vi "Poll For Jobs.vi"(8 "Error In":errorcluster, 10 "Job Queue WaitTime (5)":i32=5, 11 "VIChallenge Config in":T2) -> (0 "Error Ou":errorcluster, 2 "Worker State":T1, 3 "VIChallenge Config out":T2)   [LabVIEW 2013, in "VIChallenge.lvlib"]
uses:
  <vilib>/LabVIEW Hacker/VIChallenge/VIChallenge.lvlib
  <vilib>/LabVIEW Hacker/VIChallenge/Private/Type Defs/VIChallenge Config.ctl
  <vilib>/National Instruments/NI Amazon Web Services (AWS) Toolkit for LabVIEW/SQS/VI Source/AWS SQS Class/AWS_SQS.lvclass
  <vilib>/National Instruments/NI Amazon Web Services (AWS) Toolkit for LabVIEW/AWS Core Lib/VI Source/Typedefs/AWS_AWS Credentials.ctl
  <vilib>/LabVIEW Hacker/VIChallenge/Private/Type Defs/JSON_job.ctl
  <vilib>/addons/database/Connection.llb/Conn ObjectReference.ctl
  <vilib>/LabVIEW Hacker/VIChallenge/Private/Grader/Type Defs/Challenge.ctl
  <vilib>/LabVIEW Hacker/VIChallenge/Public/Worker State.ctl
  <vilib>/National Instruments/NI Amazon Web Services (AWS) Toolkit for LabVIEW/SQS/VI Source/Public Typedefs/AWS_SQS ReceiveMessage.ctl
  <vilib>/National Instruments/NI Amazon Web Services (AWS) Toolkit for LabVIEW/SQS/VI Source/Public Typedefs/AWS_SQS Queue Name and Account Number.ctl
  <vilib>/National Instruments/NI Amazon Web Services (AWS) Toolkit for LabVIEW/SQS/VI Source/AWS_SQS.lvlib
  <vilib>/National Instruments/NI Amazon Web Services (AWS) Toolkit for LabVIEW/AWS Core Lib/VI Source/AWS_Core.lvlib
  <vilib>/addons/database/NI_Database_API.lvlib
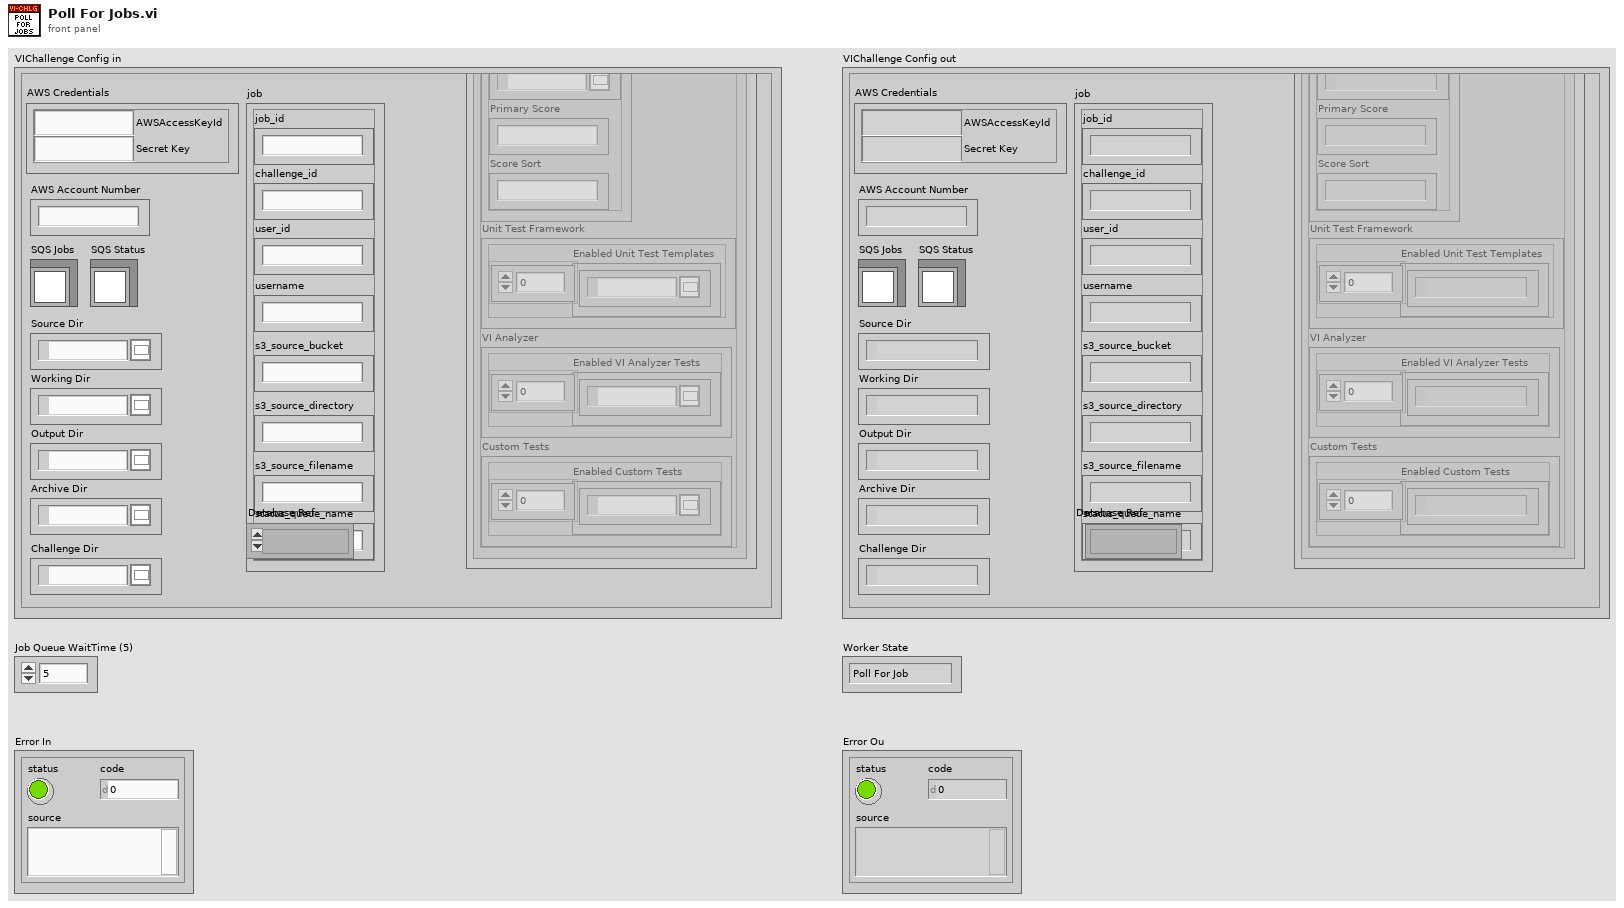
[diagram p1: front panel]
types:
  T1 = typedef "VIChallenge.lvlib/Worker State.ctl" = enum16{"Poll For Job", "Get Source", "Grade", "Notify User"}
  T2 = typedef "VIChallenge.lvlib/VIChallenge Config.ctl" = cluster{"AWS Credentials":T3, "AWS Account Number":string, "SQS Jobs":refnum<class "AWS_SQS.lvclass">, "SQS Status":refnum<class "AWS_SQS.lvclass">, "Source Dir":path, "Working Dir":path, "Output Dir":path, "Archive Dir":path, "job":T4, "Database Ref":T5, "Challenge Dir":path, "Challenges":T6[]}
  T3 = typedef "AWS_Core.lvlib/AWS_AWS Credentials.ctl" = cluster{"AWSAccessKeyId":string, "Secret Key":string}
  T4 = typedef "VIChallenge.lvlib/JSON_job.ctl" = cluster{"job_id":string, "challenge_id":string, "user_id":string, "s3_source_bucket":string, "s3_source_directory":string, "s3_source_filename":string, "status_queue_name":string, "username":string}
  T5 = typedef "NI_Database_API.lvlib/Conn ObjectReference.ctl" = refnum<k1>
  T6 = typedef "VIChallenge.lvlib/Challenge.ctl" = cluster{"General":cluster{"Challenge Id":i32, "Template Path":path, "Solution Path":path, "Primary Score":string, "Score Sort":string}, "Unit Test Framework":cluster{"Enabled Unit Test Templates":path[]}, "VI Analyzer":cluster{"Enabled VI Analyzer Tests":path[]}, "Custom Tests":cluster{"Enabled Custom Tests":path[]}}
  T7 = typedef "AWS_SQS.lvlib/AWS_SQS ReceiveMessage.ctl" = cluster{"AttributeNames":string[], "MaxNumberOfMessages":i32, "VisibilityTimeout":i32, "WaitTimeSeconds":i32}
  T8 = typedef "AWS_SQS.lvlib/ReceiveMesageResult.ctl" = cluster{"Body":string, "MD5OfBody":string, "MessageId":string, "ReceiptHandle":string, "Attributes":cluster{"AttributeName":string, "AttributeValue":string}[]}
  T9 = typedef "AWS_SQS.lvlib/AWS_SQS Queue Name and Account Number.ctl" = cluster{"QueueName":string, "Account Number":string}
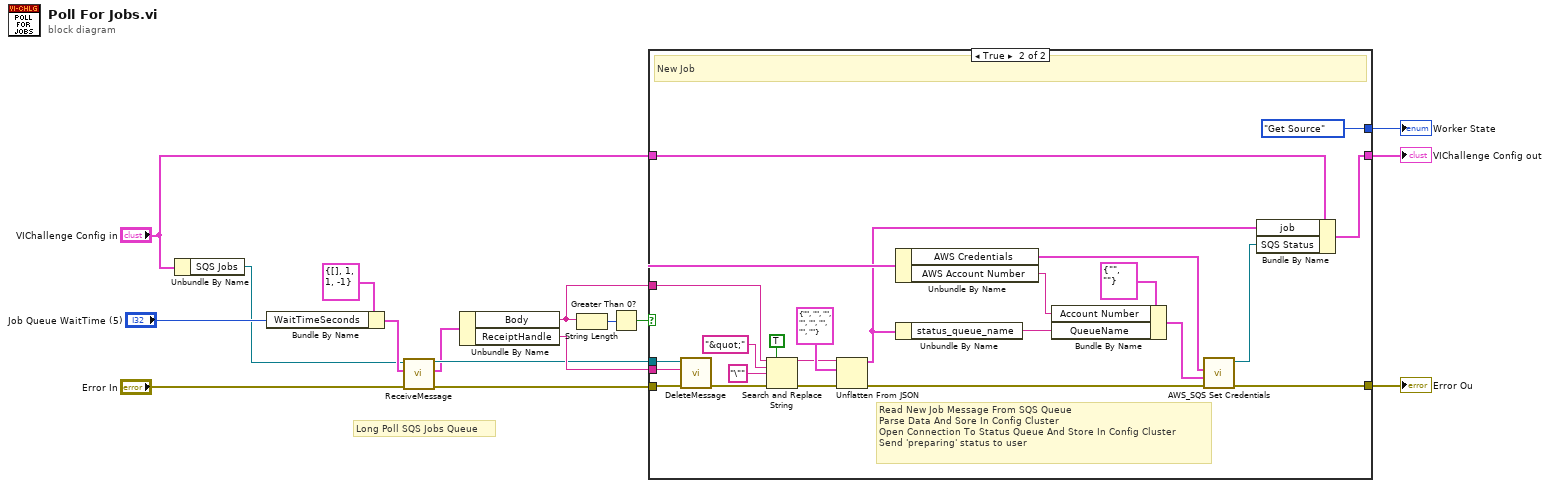
[diagram p0: block diagram]
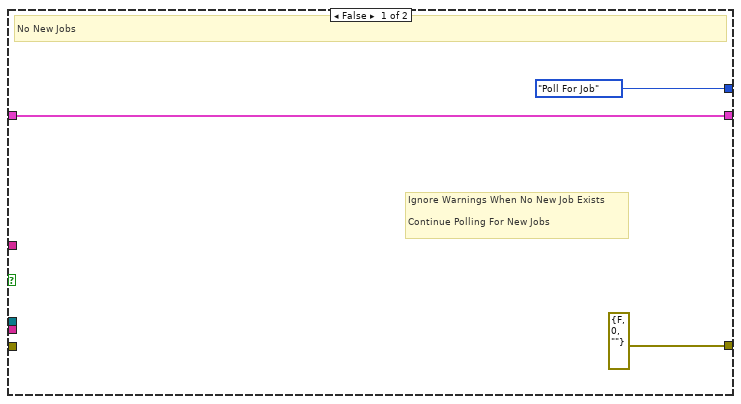
[diagram p2: hidden frame]
diagram:
  # "Long Poll SQS Jobs Queue"
  n1 = Unbundle By Name("VIChallenge Config in") -> ("SQS Jobs"=w1:refnum<class "AWS_SQS.lvclass">)
  n2 = Bundle By Name(cluster=T7 {"AttributeNames"=[], "MaxNumberOfMessages"=1, "VisibilityTimeout"=1, "WaitTimeSeconds"=-1} ("ReceiveMessage Parameters"), "WaitTimeSeconds"="Job Queue WaitTime (5)") -> (w5:T7)
  n3 = call <vilib>:"ReceiveMessage.vi"("error in (no error)"="Error In", "ReceiveMessage Parameters"=w5, "AWS_SQS.lvlib:AWS_SQS.lvclass"=w1) -> ("error out"=w9:errorcluster, "Message"=w6:T8, "AWS_SQS.lvlib:AWS_SQS.lvclass"=w12:refnum<class "AWS_SQS.lvclass">)  [unwired: 6 in]
  n4 = Unbundle By Name(w6) -> ("Body"=w14:string, "ReceiptHandle"=w13:string)
  n5 = String Length(string=w14) -> (length=w7:i32)
  n6 = Greater Than 0?(x=w7) -> (x > 0?=w8:bool)
  n7 = case shown="True" w8 {
    tunnel: w9 -> [_ w41]
    tunnel: [errorcluster {"status"=FALSE, "code"=0, "source"=""} ("Error Out") w21] -> w10
    tunnel: [Worker_State."Poll For Job" ("Worker State") Worker_State."Get Source" ("Worker State")] -> w11
    tunnel: w12 -> [_ w40]
    tunnel: w13 -> [_ w39]
    tunnel: w14 -> [_ w34]
    tunnel: "VIChallenge Config in" -> [w17 w28]
    tunnel: [w17 w30] -> w16
    frame False {
      # "Ignore Warnings When No New Job Exists\n\nContinue Polling For New Jobs"
      # "No New Jobs"
    }
    frame True {
      # "Read New Job Message From SQS Queue\nParse Data And Sore In Config Cluster\nOpen Connection To Status Queue And Store In Config Cluster\nSend 'preparing' status to user"
      # "New Job"
      n8 = call <vilib>:"DeleteMessage.vi"("error in (no error)"=w41, "ReceiptHandle"=w39, "AWS_SQS.lvlib:AWS_SQS.lvclass"=w40) -> ("error out"=w32:errorcluster)  [unwired: 5 in, 3 out]
      n9 = Search and Replace String(replace all?=TRUE ("replace all? (F)"), input string=w34, search string="&quot;", replace string="\"" ("replace string (\"\")"), error in=w32) -> (result string=w31:string, error out=w33:errorcluster)  [unwired: 3 in, 2 out]
      n10 = Unflatten From JSON(JSON string=w31, type and defaults=T4 {"job_id"="", "challenge_id"="", "user_id"="", "s3_source_bucket"="", "s3_source_directory"="", "s3_source_filename"="", "status_queue_name"="", "username"=""} ("job"), error in (no error)=w33) -> (value=w26:T4, error out=w29:errorcluster)  [unwired: 4 in]
      n11 = Unbundle By Name(w28) -> ("AWS Credentials"=w22:T3, "AWS Account Number"=w24:string)
      n12 = Unbundle By Name(w26) -> ("status_queue_name"=w25:string)
      n13 = Bundle By Name(cluster=T9 {"QueueName"="", "Account Number"=""} ("Queue Name and Account Number"), "Account Number"=w24, "QueueName"=w25) -> (w23:T9)
      n14 = call <vilib>:"AWS_SQS Set Credentials.vi"("error in (no error)"=w29, "Queue Name and Account Number"=w23, "AWS Credentials"=w22) -> ("error out"=w21:errorcluster, "AWS_SQS out"=w20:refnum<class "AWS_SQS.lvclass">)  [unwired: 7 in]
      n15 = Bundle By Name(cluster=w28, "job"=w26, "SQS Status"=w20) -> (w30:T2)
    }
  }
  "VIChallenge Config out" <- w16
  "Worker State" <- w11
  "Error Ou" <- w10
